vi "ABCtoDQ_noSine_src.vi"(5 "sinx":sgl, 7 "cosx":sgl, 9 "C":sgl, 10 "B":sgl, 11 "A":sgl) -> (0 "beta":sgl, 1 "alpha":sgl, 2 "quadrature":sgl, 3 "direct":sgl)   [LabVIEW 2015]
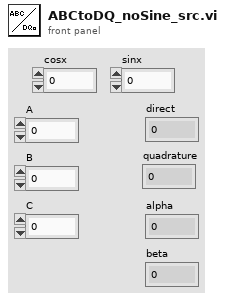
[diagram p1: front panel]
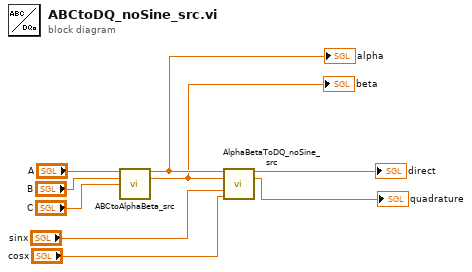
[diagram p0: block diagram]
diagram:
  n1 = call "ABCtoAlphaBeta_src.vi"("A"="A", "B"="B", "C"="C") -> ("alpha"=w9:sgl, "beta"=w8:sgl)  [unwired: 11 in]
  "alpha" <- w9
  "beta" <- w8
  n2 = call "AlphaBetaToDQ_noSine_src.vi"("alpha"=w9, "beta"=w8, "sinx"="sinx", "cosx"="cosx") -> ("direct"=→"direct":sgl, "quadrature"=→"quadrature":sgl)  [unwired: 10 in]
